vi "GOOP_ColorToARGB.vi"(0 "Color":u32, 11 "error in":errorcluster) -> (4 "A":u8, 6 "R":u8, 8 "G":u8, 10 "B":u8, 15 "error out":errorcluster)   [LabVIEW 2020]
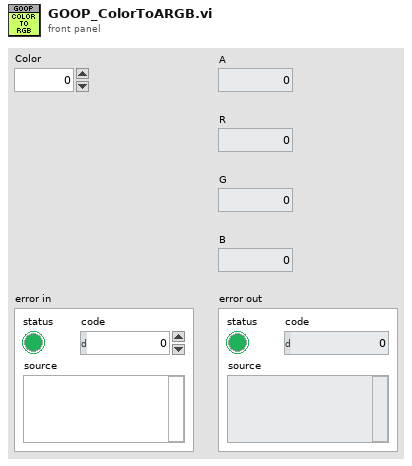
[diagram p1: front panel]
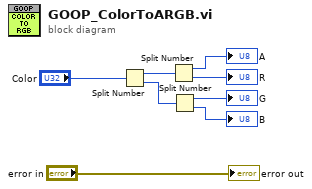
[diagram p0: block diagram]
diagram:
  n1 = Split Number(x="Color") -> (hi(x)=w6:u16, lo(x)=w5:u16)
  n2 = Split Number(x=w6) -> (hi(x)=→"A":u8, lo(x)=→"R":u8)
  n3 = Split Number(x=w5) -> (hi(x)=→"G":u8, lo(x)=→"B":u8)
  "error out" <- "error in"
